vi "READ - File.vi"(0 "reference in":refnum<class "HeadAcousticHDF.lvclass">, 5 "error in (no error)":errorcluster, 7 "Path - READ":path, 9 "Channel Selected (0=ALL)":i32) -> (14 "reference out":refnum<class "HeadAcousticHDF.lvclass">, 19 "error out":errorcluster)   [LabVIEW 2022 SP3, in "HeadAcousticHDF.lvclass"]
uses:
  HeadAcousticHDF.lvclass
  API/GSwFormDSP_class/functions/Attribute List.ctl
  <vilib>/Platform/storage/lvStorage.llb/_openStorageWithRootAutoDetect.vi
  <vilib>/Platform/storage/lvStorage.llb/xStorage/xStorageSupp/ErrorOut.vi
  <vilib>/Platform/storage/lvStorage.llb/_queryPropPoly.vi
  <vilib>/Platform/storage/lvStorage.llb/_queryPropString.vi
  <vilib>/Platform/storage/lvStorage.llb/_queryGenericObjects.vi
  <vilib>/Platform/storage/lvStorage.llb/_loadAllWaveform.vi
  <vilib>/Platform/storage/Storage.llb/Get Object Info.vi
  <vilib>/Platform/storage/Storage.llb/__closeStorageFromObject.vi
  <vilib>/Platform/storage/lvStorage.llb/xStorage/Open Data Storage/Open Data Storage.xnode
  <vilib>/Platform/storage/lvStorage.llb/xStorage/Read Data/Read Data.xnode
  <vilib>/Platform/storage/lvStorage.llb/xStorage/Close Data Storage/Close Data Storage.xnode
  API/GSwFormDSP_class/GSwFormDSP.lvclass
  API/Generic Utilities_class/Generic Utilities.lvclass
  <vilib>/Platform/storage/lvStorage.llb/_loadAllDdt.vi
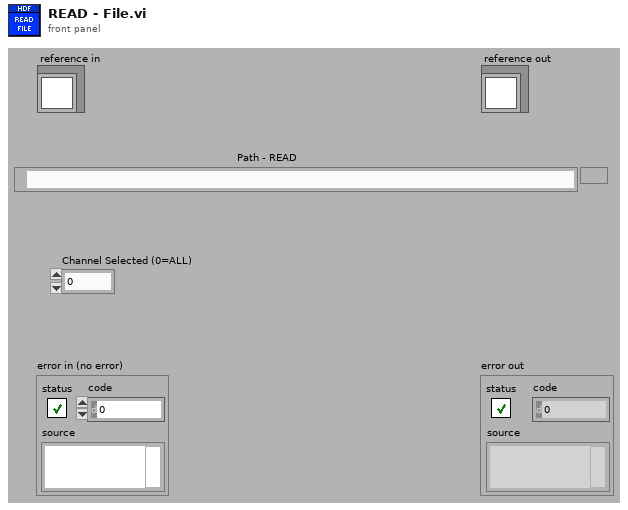
[diagram p1: front panel]
types:
  T1 = typedef "GSwFormDSP.lvclass/Attribute List.ctl" = string
  T2 = enum16{"open", "open or create", "create or replace", "create", "open (read only)"}
  T3 = enum16{"UPDATE", "READ", "QUERY", "CREATE CHILD", "CREATE", "CONNECT", "DISCONNECT"}
  T4 = typedef "HeadAcousticHDF.lvclass/ObjectAttributesRef.ctl" = refnum<data-value>
  T5 = typedef "HeadAcousticHDF.lvclass/ObjectAttributes.ctl" = cluster{"Time Data":refnum<class "GSwFormDSP.lvclass">, "Data Plugin Name":string, "Additional Data Plugin Name":string, "New Time Data Obj?":bool}
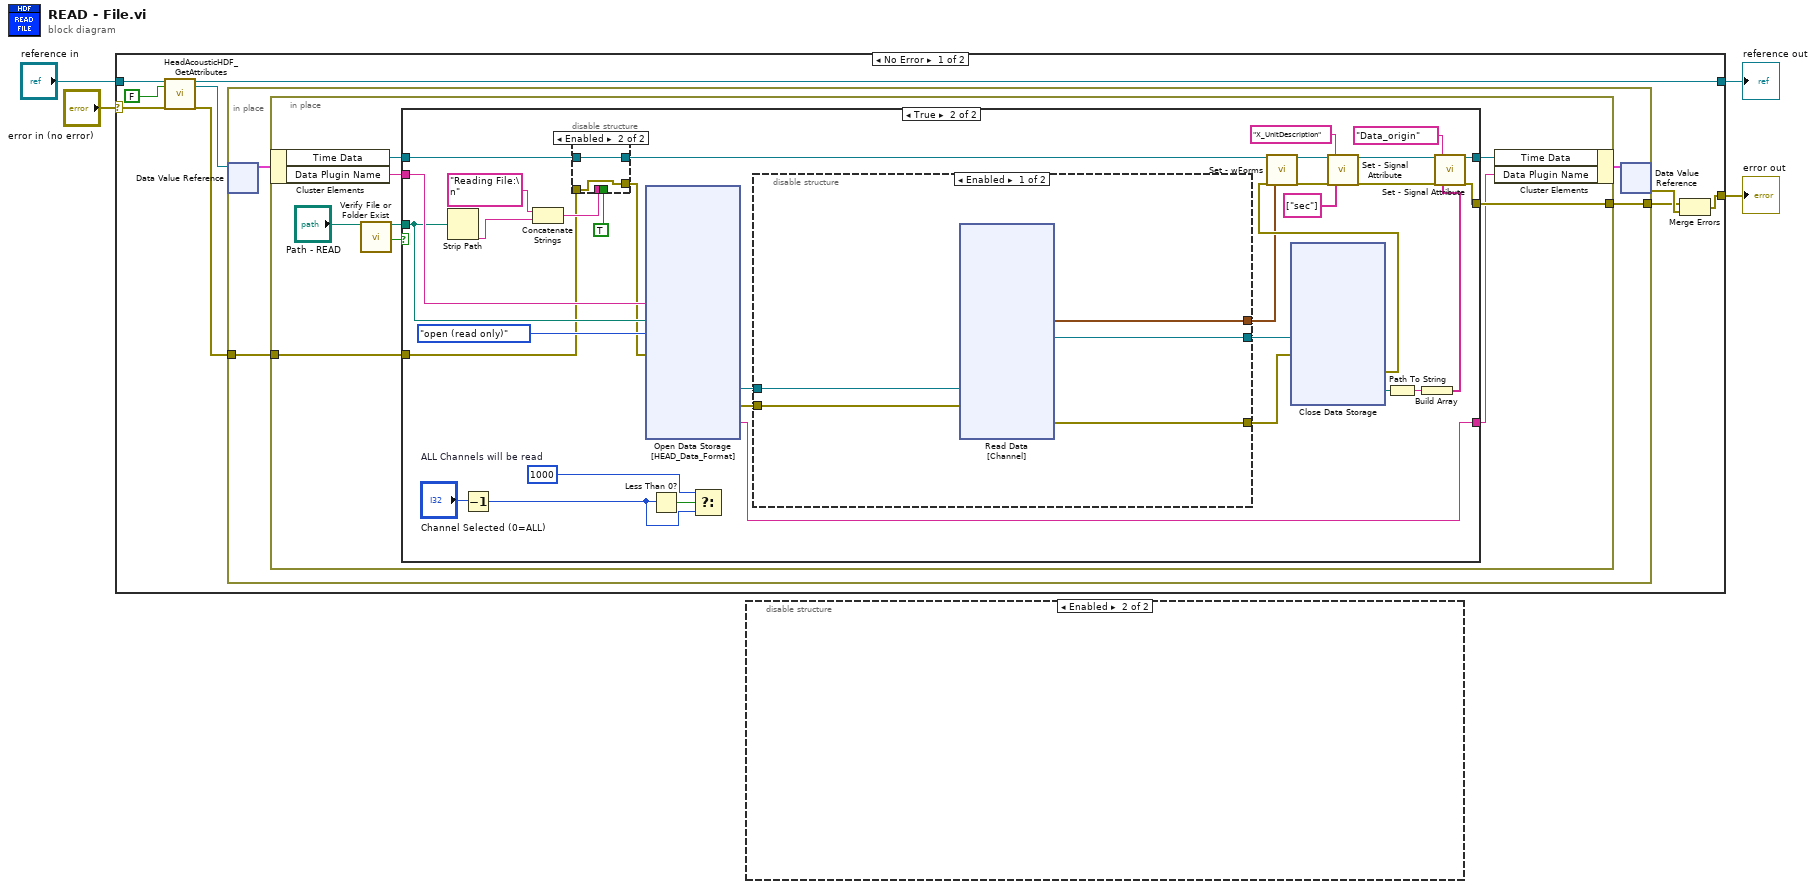
[diagram p0: block diagram]
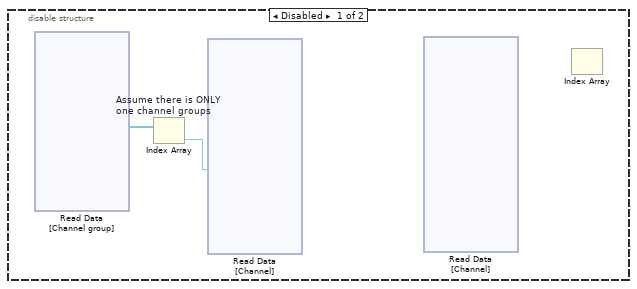
[diagram p2: hidden frame]
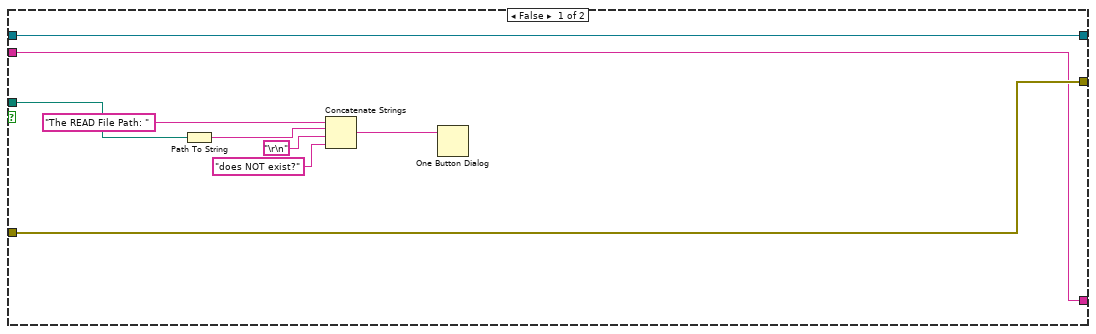
[diagram p3: hidden frame]
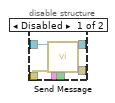
[diagram p4: hidden frame]
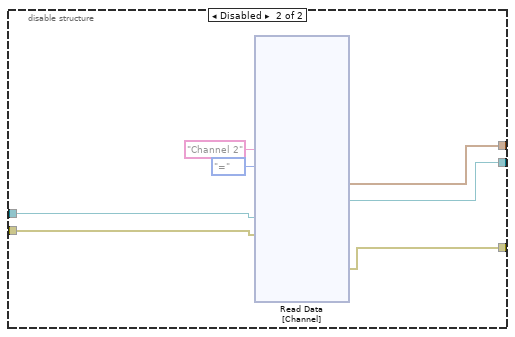
[diagram p5: hidden frame]
diagram:
  n1 = case shown="No Error" "error in (no error)" {
    selector: "error in (no error)" -> [w8 w143]
    tunnel: [w13 w143] -> w3
    tunnel: [w7 w142] -> w1
    tunnel: "reference in" -> [w10 w142]
    frame No Error {
      n2 = call "HeadAcousticHDF_GetAttributes.vi"("reference in"=w10, "return data? (T)"=FALSE, "error in (no error)"=w8) -> ("reference out"=w7:refnum<class "HeadAcousticHDF.lvclass">, "attributes ref"=w6:T4, "error out"=w5:errorcluster)  [unwired: 13 in, 1 out]
      n3 = in-place {
        in-place-border: [w14] -> w11
        in-place-border: w5 -> [w15]
        n4 = in-place-dvr #1(w6) -> (w16:T5)  [unwired: 1 out]
        n5 = in-place {
          in-place-border: w15 -> [w21]
          in-place-border: [w20] -> w14
          n6 = in-place-cluster #2(w16) -> ("Time Data"=w22:refnum<class "GSwFormDSP.lvclass">, "Data Plugin Name"=w19:string)
          n7 = call "Verify File or Folder Exist.vi"("path"="Path - READ") -> ("dup path"=w26:path, "file or folder exists?"=w25:bool)  [unwired: 16 in, 1 out]
          n8 = case shown="True" w25 {
            tunnel: w22 -> [w35 w40]
            tunnel: [w35 w68] -> w23
            tunnel: w26 -> [w33 w39]
            tunnel: w21 -> [w34 w38]
            tunnel: [w34 w69] -> w20
            tunnel: w19 -> [w27 w67]
            tunnel: [w27 w57] -> w18
            frame False {
              n9 = Path To String(path=w33) -> (string=w31:string)
              n10 = Concatenate Strings("The READ File Path: ", w31, "\r\n", "does NOT exist?") -> (w28:string)
              n11 = One Button Dialog(message=w28) -> ()  [unwired: 1 in, 1 out]
            }
            frame True {
              w58 = 1000  # ALL Channels will be read
              n12 = Strip Path(path=w39) -> (name=w43:string)  [unwired: 1 out]
              n13 = Decrement(x="Channel Selected (0=ALL)") -> (x-1=w59:i32)
              n14 = Concatenate Strings("Reading File:\n", w43) -> (w42:string)
              n15 = disable-structure shown="Enabled" {
                disable-tunnel: w42 -> [w75 _]
                disable-tunnel: TRUE ("Make Cursor Busy?") -> [w74 _]
                disable-tunnel: w40 -> [w73 w77]
                disable-tunnel: w38 -> [w72 w76]
                disable-tunnel: [w71 w76] -> w37
                disable-tunnel: [w70 w77] -> w36
                frame Disabled {
                  n16 = call-dynamic "Send Message.vi"("reference in"=w73, "error in (no error)"=w72, "Message (\"\" closes the window)"=w75, "Make Cursor Busy?"=w74) -> ("reference out"=w70:refnum<class "GSwFormDSP.lvclass">, "error out"=w71:errorcluster)  [unwired: 14 in]
                }
                frame Enabled {
                }
              }
              n17 = xnode "Open Data Storage\n[HEAD_Data_Format]"("DataPlugin name"=w67, "file path"=w39, "function (open:0)"=T2."open (read only)", "error in (no error)"=w37) -> ("storage refnum (file)"=w55:refnum<k20>, "error out"=w56:errorcluster, "DataPlugin name out"=w57:string)  [unwired: 1 in]
              n18 = Less Than 0?(x=w59) -> (x < 0?=w60:bool)
              n19 = Select(t=w58, s=w60, f=w59) -> ()  [unwired: 1 out]
              n20 = disable-structure shown="Enabled" {
                disable-tunnel: [w82 w104] -> w65
                disable-tunnel: [w81 w101] -> w64
                disable-tunnel: [w80 w102] -> w62
                disable-tunnel: w56 -> [w79 w103]
                disable-tunnel: w55 -> [w78 w105]
                frame Enabled {
                  n21 = xnode "Read Data\n[Channel]"("storage refnum (file)"=w78, "error in"=w79) -> ("Signal"=w80:waveform(dbl)[], "storage refnum (file) out"=w81:refnum<k20>, "error out"=w82:errorcluster)  [unwired: 2 in, 1 out]
                }
                frame Disabled {
                  n22 = xnode "Read Data\n[Channel]"("Name"="Channel 2", "Comparison (=)"=enum16{"=", "!=", ">", "<", ">=", "<="}."=", "storage refnum (file)"=w105, "error in"=w103) -> ("Signal"=w102:waveform(dbl)[], "storage refnum (file) out"=w101:refnum<k20>, "error out"=w104:errorcluster)  [unwired: 2 in, 1 out]
                }
              }
              n23 = xnode "Close Data Storage\n"("storage refnum (file)"=w64, "error in (no error)"=w65) -> ("error out"=w63:errorcluster, "file path"=w54:path)
              n24 = call "Set - wForms.vi"("reference in"=w36, "error in (no error)"=w63, "wForms"=w62) -> ("reference out"=w48:refnum<class "GSwFormDSP.lvclass">, "error out"=w47:errorcluster)  [unwired: 15 in]
              n25 = call-dynamic "Set - Signal Attribute.vi"("reference in"=w48, "error in (no error)"=w47, "wForm Attributes"=T1 "X_UnitDescription", "Attribute"=string[] ["sec"]) -> ("reference in"=w49:refnum<class "GSwFormDSP.lvclass">, "error out"=w50:errorcluster)  [unwired: 14 in]
              n26 = Path To String(path=w54) -> (string=w53:string)
              n27 = Build Array(w53) -> (w52:string[])
              n28 = call-dynamic "Set - Signal Attribute.vi"("reference in"=w49, "error in (no error)"=w50, "wForm Attributes"=T1 "Data_origin", "Attribute"=w52) -> ("reference in"=w68:refnum<class "GSwFormDSP.lvclass">, "error out"=w69:errorcluster)  [unwired: 14 in]
            }
          }
          n29 = in-place-cluster #2("Time Data"=w23, "Data Plugin Name"=w18) -> (w17:T5)
        }
        n30 = in-place-dvr #1(w17) -> (w12:errorcluster)  [unwired: 1 out]
      }
      n31 = Merge Errors(w11, w12) -> (w13:errorcluster)
    }
    frame Error {
    }
  }
  "error out" <- w3
  "reference out" <- w1
  n32 = disable-structure shown="Enabled" {
    frame Disabled {
      n33 = xnode "Read Data\n[Channel group]"() -> ("storage refnums (channel group)"=w144:refnum<k20>[])  [unwired: 2 in, 2 out]
      n34 = Index Array "Assume there is ONLY one channel groups"(array=w144) -> (element=w145:refnum<k20>)  [unwired: 1 in]
      n35 = xnode "Read Data\n[Channel]"("storage refnum (channel group)"=w145) -> ()  [unwired: 3 in, 4 out]
      n36 = xnode "Read Data\n[Channel]"() -> ()  [unwired: 4 in, 4 out]
      n37 = Index Array() -> ()  [unwired: 2 in, 1 out]
    }
    frame Enabled {
    }
  }
